vi "pop_dialog.vi"(8 "Property":string[](array[string]), 9 "State In":T2 {"BlockNodeState"."Draw Style" items=["FunctionBlock", "ExpressVI", "Variable", "Elemental I/O", "32x32 Icon", "FunctionBlockCompact"]; "BlockNodeState"."Terminal Data"."Terminal Flags" format="%.0b"}, 10 "FirstTime":bool, 11 "Command Spec":T1) -> (1 "State Out":T2 {"BlockNodeState"."Draw Style" items=["FunctionBlock", "ExpressVI", "Variable", "Elemental I/O", "32x32 Icon", "FunctionBlockCompact"]; "BlockNodeState"."Terminal Data"."Terminal Flags" format="%.0b"}, 2 "NeedUpdate":bool)   [LabVIEW 2018]
uses:
  State.ctl
  <vilib>/BlockNodeSupport/BlockNodeState.ctl
  <vilib>/BlockNodeSupport/TerminalData.ctl
  <vilib>/picture/picture.llb/imagedata.ctl
  command_spec.ctl
  N9010A_SCPI Node.xnode
panel:
  in  "Sort Properties":u16(ring) items=["by Source File Order", "by Property Name", "by SCPI Command"]
  in  "Available Properties Tree":string[](tree)
  in  "Cancel Button":bool
  out "Selected Cmd Pool":string[](array[string])
  out "Available Cmd Pool":string[](array[string])
  in  "Search Within Available Properties":string
  out "Property Help":string
  out "Delete Array":i32[](array[numeric])
  in  "OK Button":bool
  in  "Remove":bool caption="Previous Button"
  in  "Add":bool
  in  "Selected Properties":i32[](listbox)
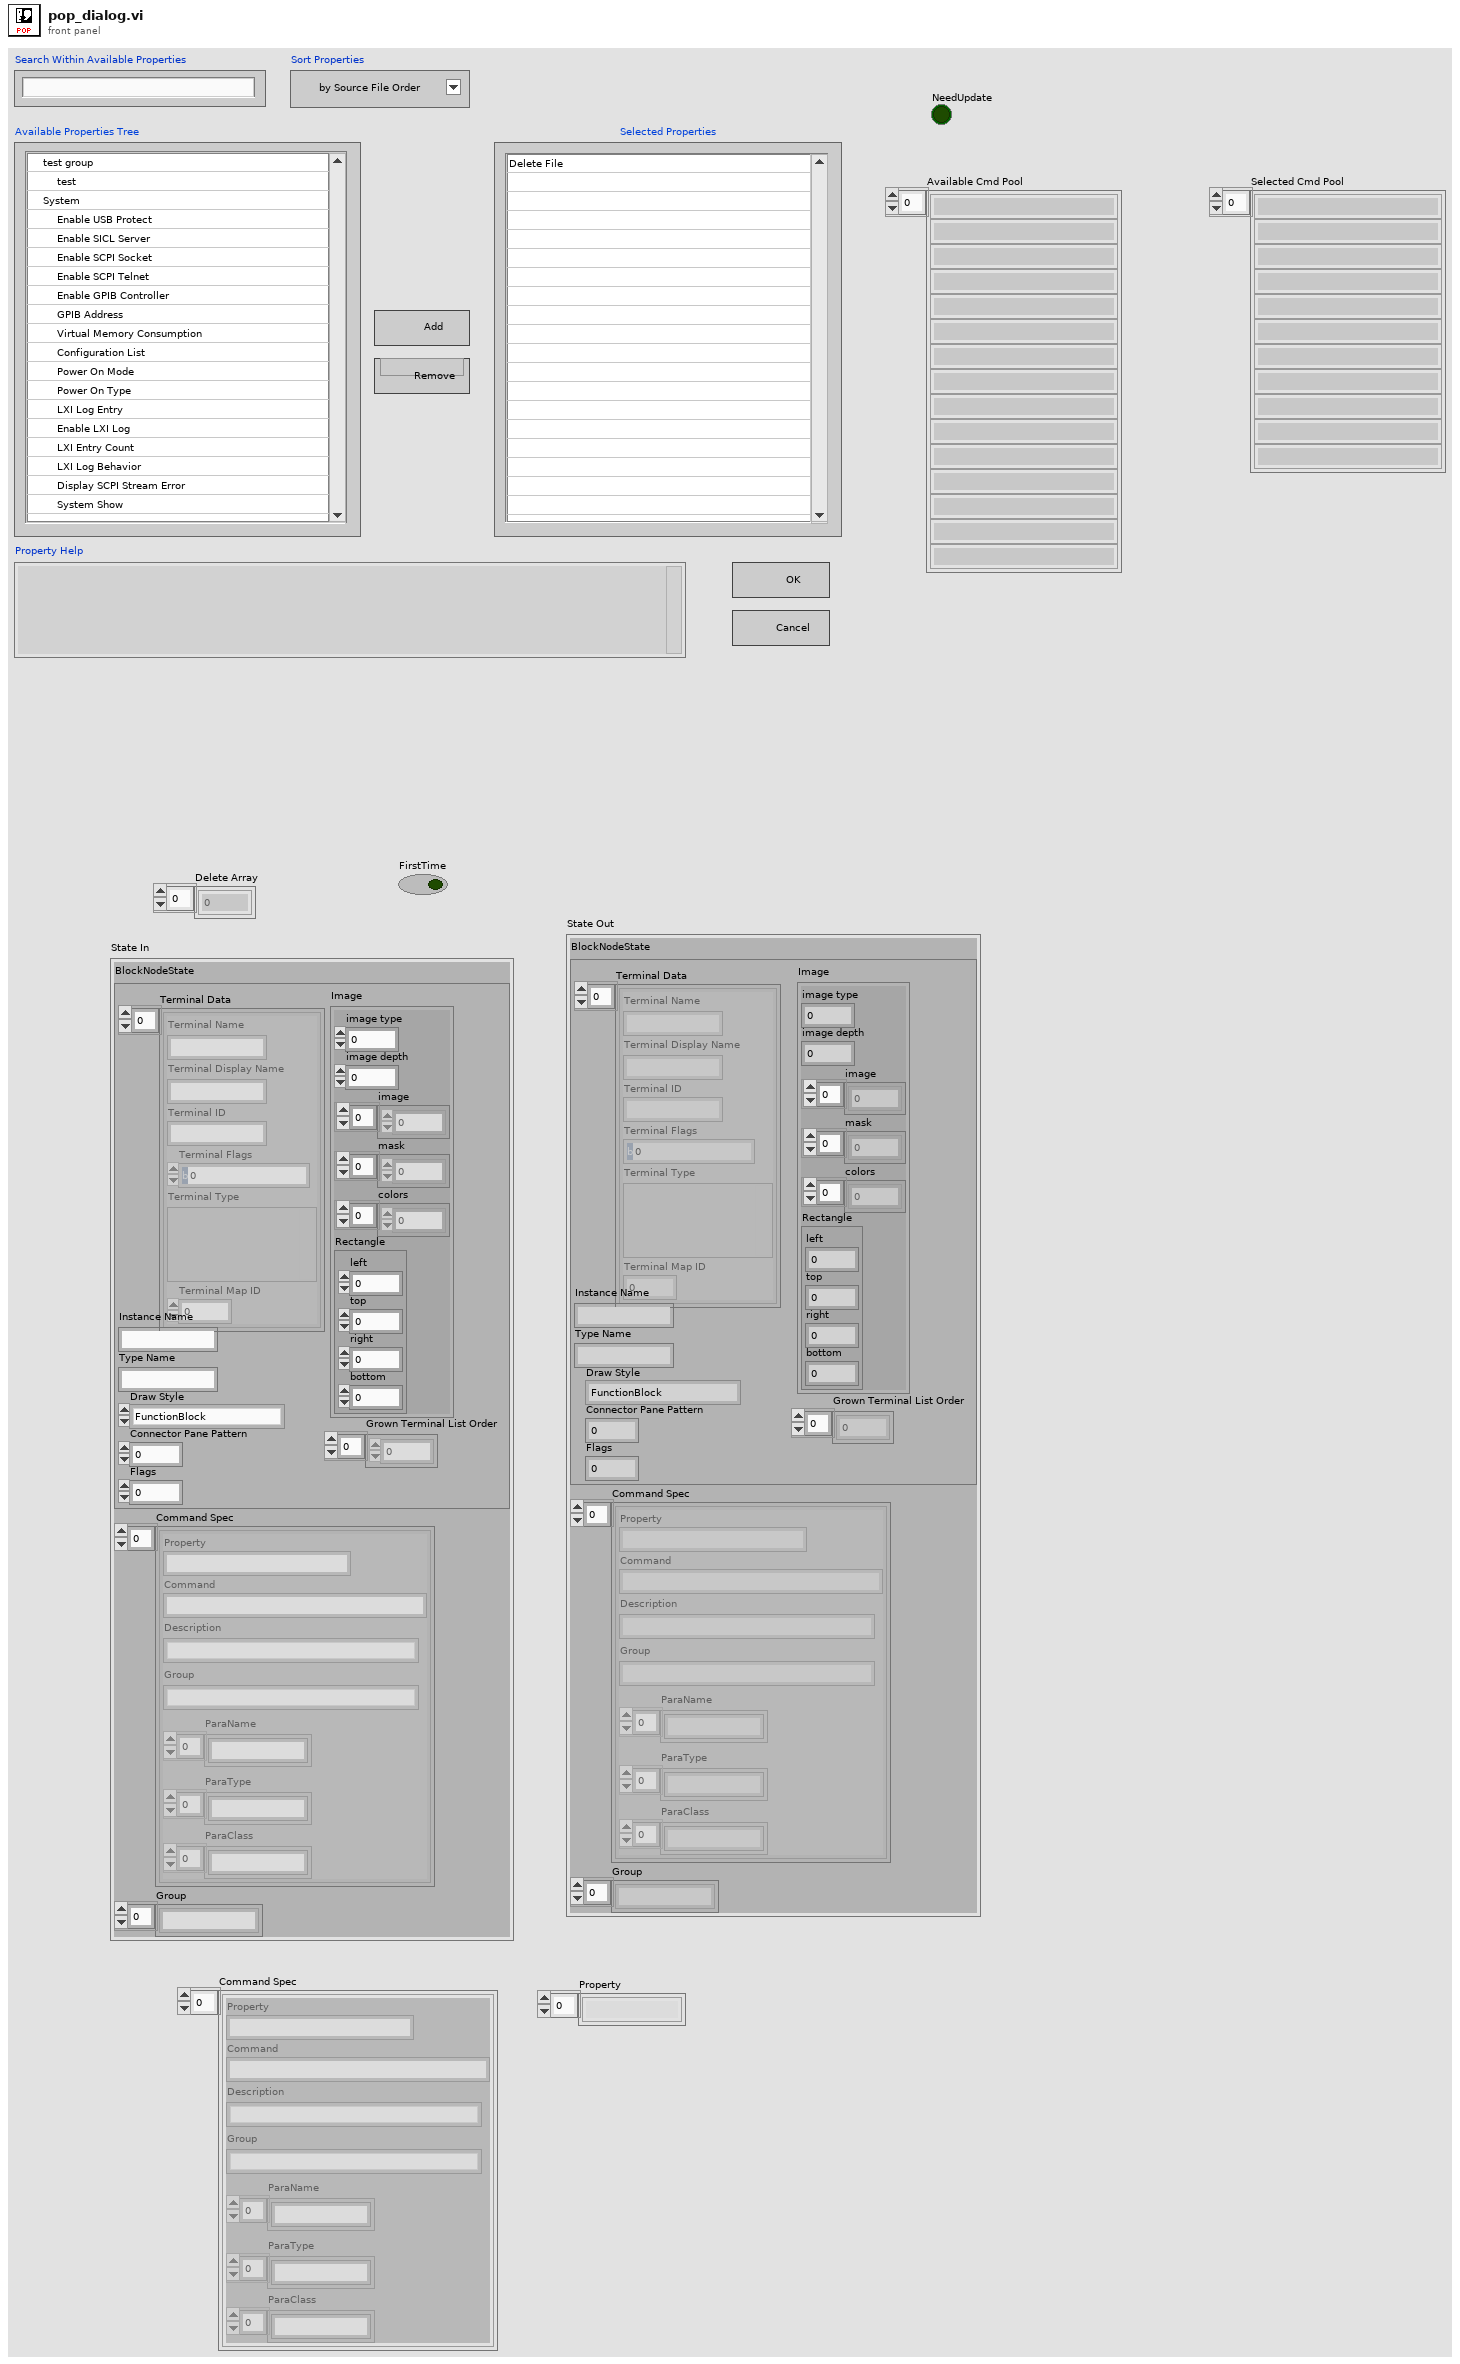
[diagram p1: front panel]
types:
  T1 = typedef "command_spec.ctl" = cluster{"Property":string, "Command":string, "Description":string, "Group":string, "ParaName":string[], "ParaType":string[], "ParaClass":string[]}[]
  T2 = typedef "N9010A_SCPI Node.xnode/State.ctl" = cluster{"BlockNodeState":T3, "Command Spec":T1, "Group":string[]}
  T3 = typedef "BlockNodeState.ctl" = cluster{"Terminal Data":T4[], "Instance Name":string, "Type Name":string, "Draw Style":i32, "Connector Pane Pattern":i32, "Flags":i32, "Grown Terminal List Order":i32[], "Image":T5}
  T4 = typedef "TerminalData.ctl" = cluster{"Terminal Name":string, "Terminal Display Name":string, "Terminal ID":string, "Terminal Flags":i32, "Terminal Type":variant, "Terminal Map ID":i32}
  T5 = typedef "imagedata.ctl" = cluster{"image type":i32, "image depth":i32, "image":u8[], "mask":u8[], "colors":u32[], "Rectangle":cluster{"left":i16, "top":i16, "right":i16, "bottom":i16}}
  T6 = enum8{"Enabled", "Disabled", "Disabled and Grayed Out"}
  T7 = typedef "LVPoint32TypeDef.ctl" = cluster{"Horizontal":i32, "Vertical":i32}
  T8 = cluster{"Property":string, "Command":string, "Description":string, "Group":string, "ParaName":string[], "ParaType":string[], "ParaClass":string[]}
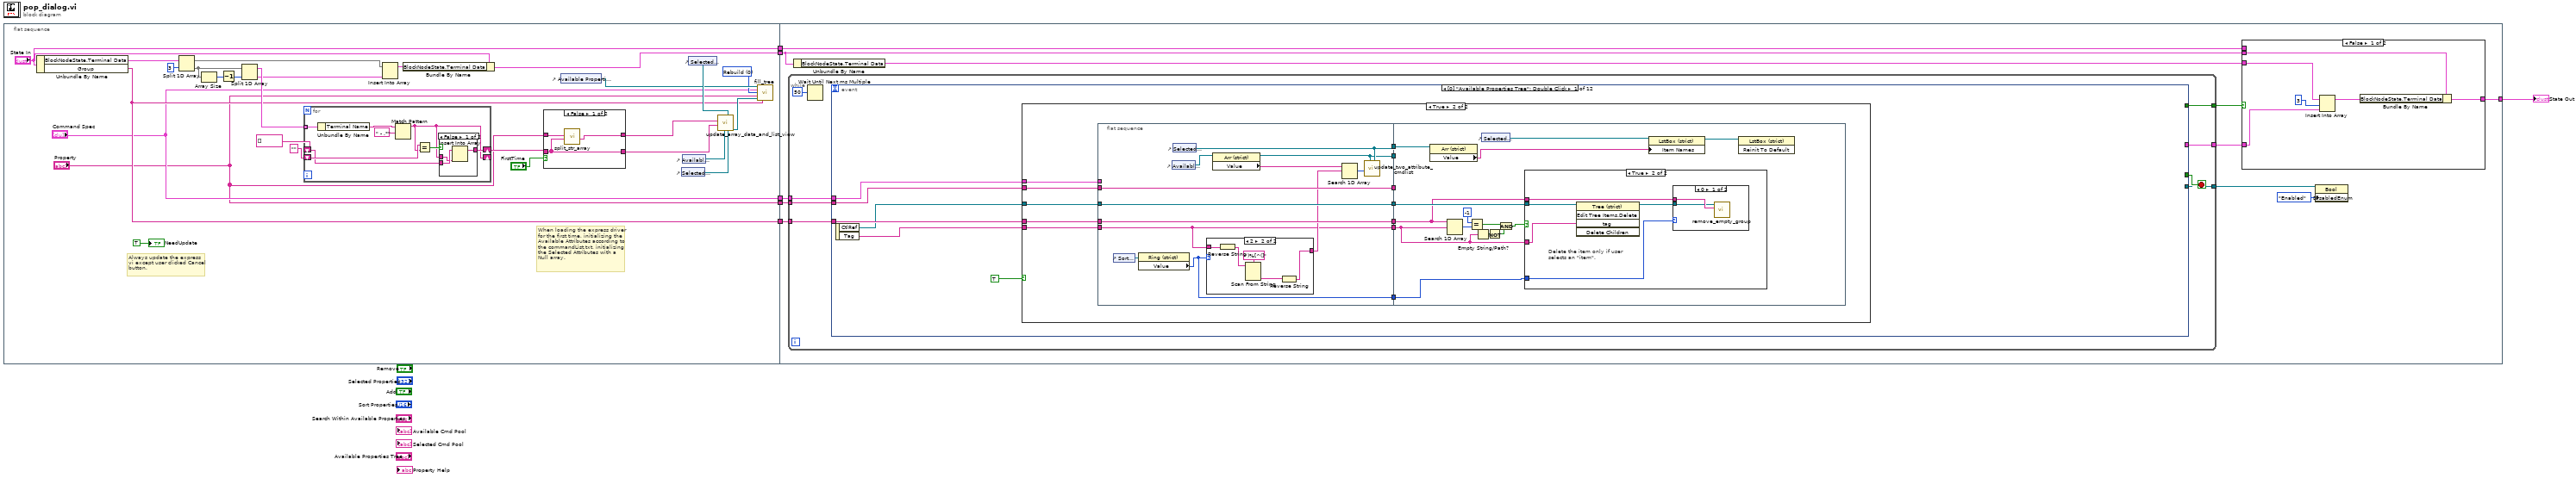
[diagram p0: block diagram]
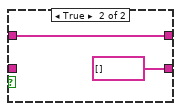
[diagram p2: hidden frame]
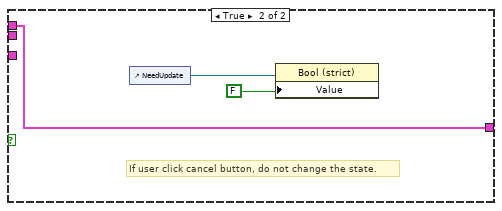
[diagram p4: hidden frame]
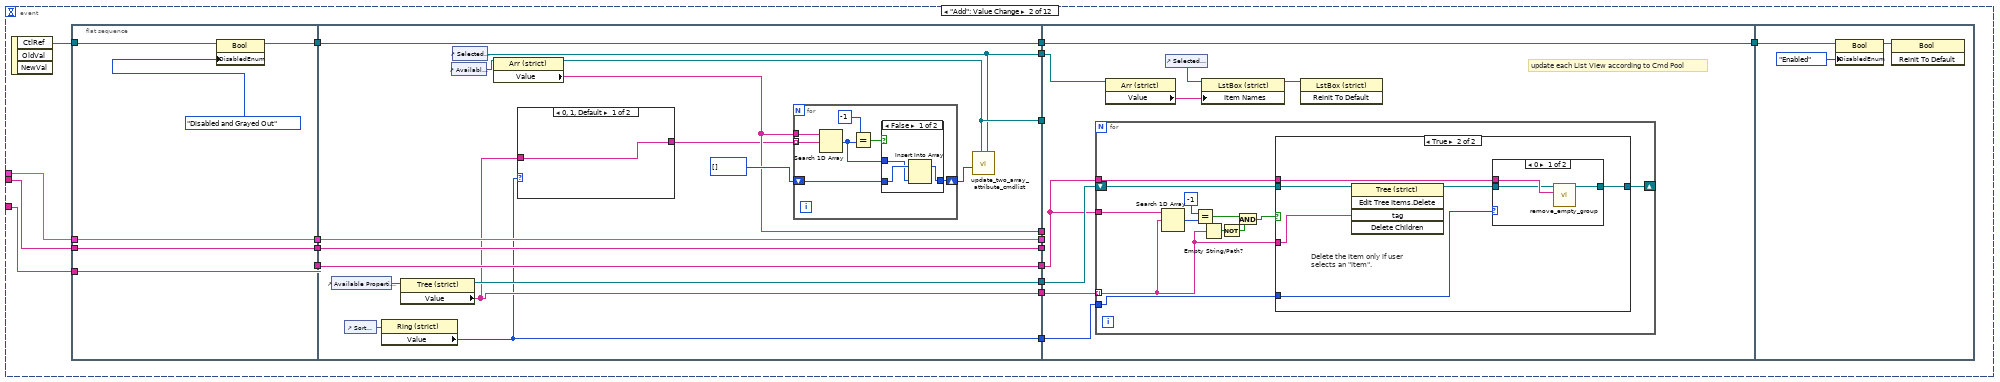
[diagram p9: hidden frame]
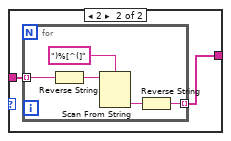
[diagram p10: hidden frame]
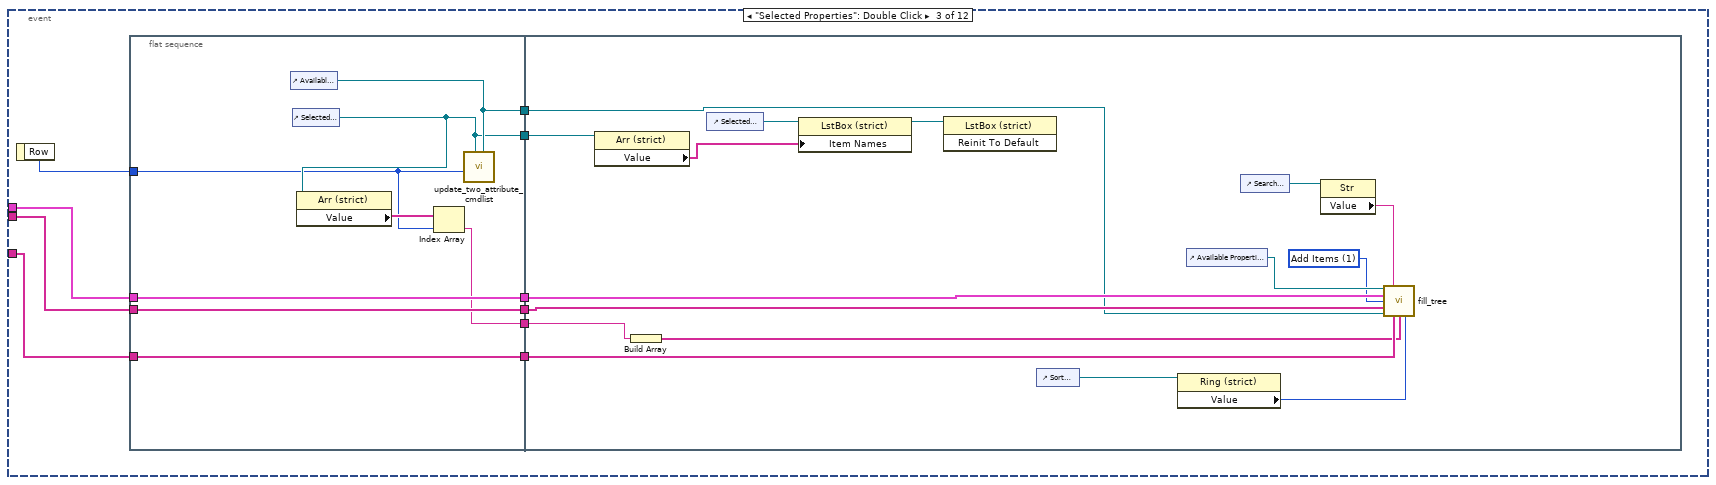
[diagram p14: hidden frame]
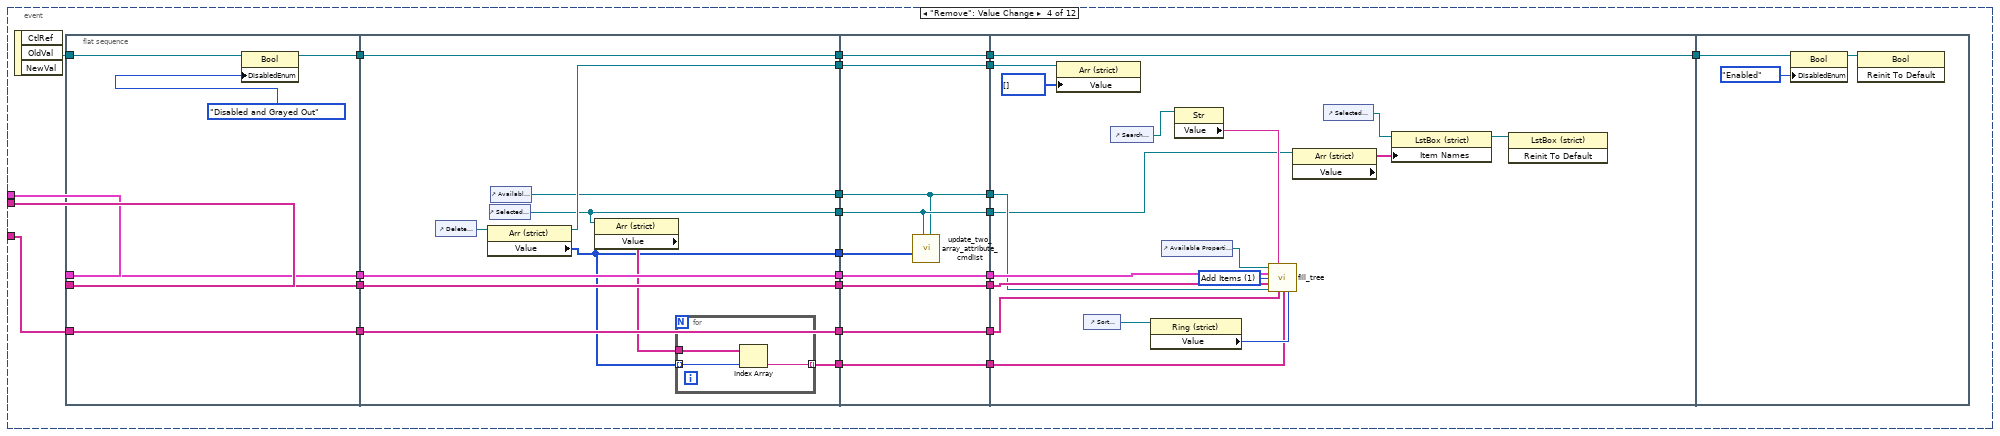
[diagram p15: hidden frame]
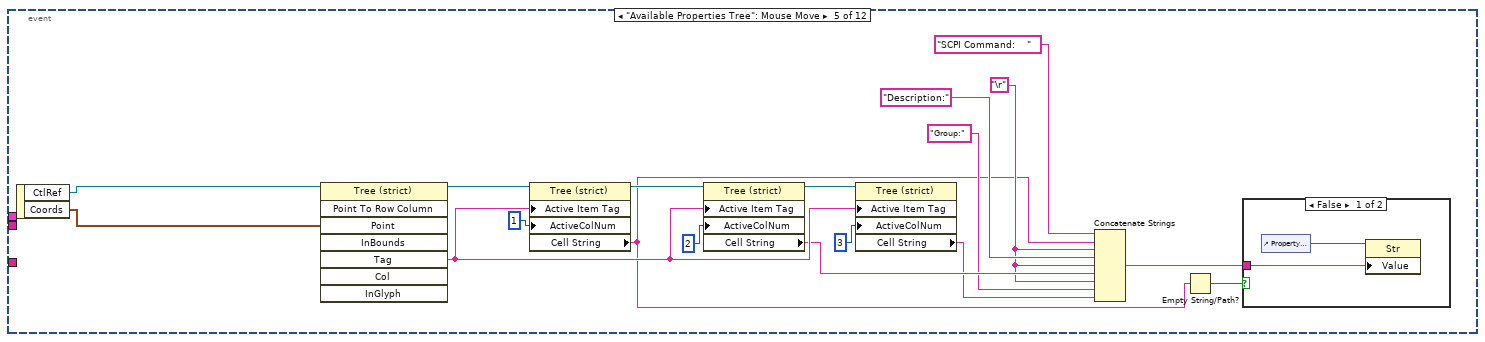
[diagram p16: hidden frame]
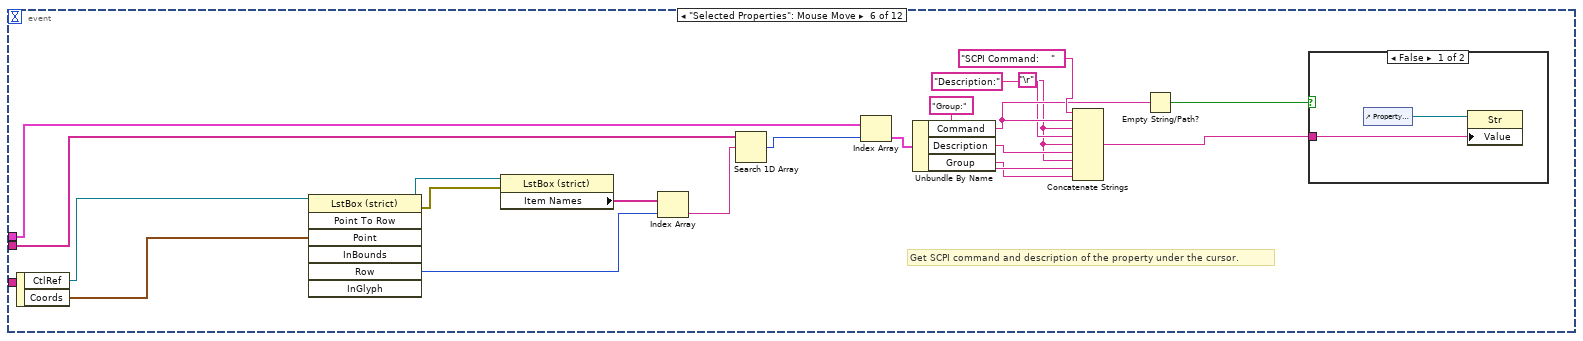
[diagram p18: hidden frame]
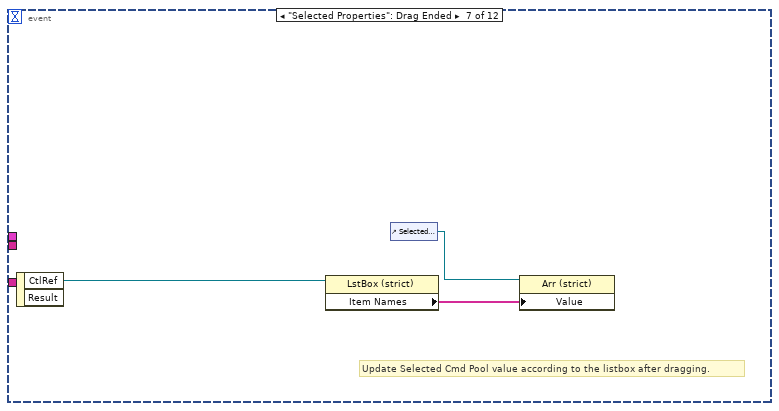
[diagram p20: hidden frame]
diagram:
  n1 = flat-sequence {
    tunnel: ["Command Spec"] -> w6
    tunnel: ["Property"] -> w5
    tunnel: [w32] -> w4
    tunnel: ["State In"] -> w2
    tunnel: [w13] -> w1
    tunnel: w6 -> [w61]
    tunnel: w5 -> [w60]
    tunnel: [w56] -> w3
    tunnel: w4 -> [w57]
    tunnel: w2 -> [w54]
    tunnel: w1 -> [w51]
    frame #0 {
      w9 = u16 0 items=["Rebuild", "Add Single"] ("Operation")
      # "Always update the express\nvi except user clicked Cancel\nbutton."
      # "When loading the express driver\nfor the first time, initializing the\nAvailable Attributes according to\nthe commandList.txt, initializing \nthe Selected Attributes with a\nNull array."
      n2 = Unbundle By Name("State In") -> ("BlockNodeState.Terminal Data"=w31:T4[], "Group"=w13:string[])
      n3 = Split 1D Array(array=w31, index=3) -> (first subarray=w24:T4[], second subarray=w28:T4[])
      n4 = Array Size(array=w28) -> (size(s)=w29:i32)
      n5 = Decrement(x=w29) -> (x-1=w27:i32)
      n6 = Split 1D Array(array=w28, index=w27) -> (first subarray=w26:T4[], second subarray=w25:T4[])
      n7 = for {
        tunnel: w26 -> [w46] mode=indexing
        shift-right: [w40] -> w10
        shift-left: string[] [] ("Array") -> [w41]
        shift-right: [w39] -> _
        shift-left: "" -> [w43]
        n8 = Unbundle By Name(w46) -> ("Terminal Name"=w44:string)
        n9 = Match Pattern(string=w44, regular expression=" - .*") -> (before substring=w39:string)  [unwired: 1 in, 3 out]
        n10 = Equal?(x=w43, y=w39) -> (x = y?=w42:bool)
        n11 = case shown="False" w42 {
          tunnel: w41 -> [w49 w50]
          tunnel: w39 -> [w48 _]
          tunnel: [w47 w50] -> w40
          frame False {
            n12 = Insert Into Array(array=w49, new element=w48) -> (w47:string[])  [unwired: 1 in]
          }
          frame True {
          }
        }
      }
      n13 = Insert Into Array(array=w24, new element=w25) -> (w23:T4[])  [unwired: 1 in]
      n14 = Bundle By Name(cluster="State In", "BlockNodeState.Terminal Data"=w23) -> (w32:T2)
      n15 = case shown="False" "FirstTime" {
        tunnel: "Property" -> [w36 w37]
        tunnel: [w34 string[] [] ("Item Names")] -> w22
        tunnel: [w35 w37] -> w16
        tunnel: w10 -> [w34 _]
        frame False {
          n16 = call "split_str_array.vi"("First  Array"=w34, "Total Array"=w36) -> ("Rest Array"=w35:string[])  [unwired: 9 in]
        }
        frame True {
        }
      }
      n17 = control-ref of="Available Properties Tree"() -> (w15:refnum<vi>)
      n18 = control-ref of="Selected Cmd Pool"() -> (w20:refnum<vi>)
      n19 = control-ref of="Available Cmd Pool"() -> (w21:refnum<vi>)
      n20 = control-ref of="Selected Properties"() -> (w19:refnum<vi>)
      n21 = call "update_array_data_and_list_view.vi"("Cmd Pool 2"=w20, "Cmd Pool 2 List View"=w19, "Cmd Pool 1"=w21, "Cmd Array 2"=w22, "Cmd Array 1"=w16) -> ("Cmd Pool 1 Ref Out"=w14:refnum<vi>)  [unwired: 6 in]
      n22 = call "fill_tree.vi"("Tree Refnum"=w15, "Command Spec"="Command Spec", "Operation"=w9, "Property"="Property", "Available Commands Pool"=w14, "Group"=w13) -> ()  [unwired: 10 in]
      "NeedUpdate" <- TRUE ("NeedUpdate")
    }
    frame #1 {
      n23 = while {
        tunnel: w61 -> [w76]
        tunnel: w60 -> [w77]
        tunnel: [w74] -> w58
        tunnel: [w73] -> w55
        tunnel: [w72] -> w53
        tunnel: w51 -> [w71]
        stop <- w78 stop-if-true
        n24 = Wait Until Next ms Multiple(millisecond multiple=u32 50) -> ()  [unwired: 1 out]
        n25 = event shown="[0] \"Available Properties Tree\": Double Click" {
          selector: _ -> [_ _ _ _ _ _ _ _ _ _ _ _]
          dyn-events: _ -> [_ _ _ _ _ _ _ _ _ _ _ _]
          timeout: _ -> [_ _ _ _ _ _ _ _ _ _ _ _]
          tunnel: [_ _ _ _ _ _ _ _ _ _ w416 "Cancel Button"] -> w78
          tunnel: w77 -> [w82 w147 w234 w287 _ w373 _ _ w391 w406 w414 _]
          tunnel: w76 -> [w83 w148 w236 w286 _ w371 _ _ w392 w407 w415 _]
          tunnel: [_ _ _ _ _ _ _ _ _ _ w412 _] -> w74
          tunnel: [_ _ _ _ _ _ _ _ _ _ _ "Cancel Button"] -> w73
          tunnel: [_ _ _ _ _ _ _ _ _ _ w417 _] -> w72
          tunnel: w71 -> [w84 w140 w233 w283 _ _ _ _ w390 w405 _ _]
          event "Available Properties Tree": Double Click {
            n26 = event-data() -> ("CtlRef"=w80:refnum<vi>, "Tag"=w81:string)  [unwired: 1 in]
            n27 = case shown="True" TRUE {
              tunnel: w84 -> [_ w89]
              tunnel: w83 -> [_ w88]
              tunnel: w82 -> [_ w87]
              tunnel: w81 -> [_ w86]
              tunnel: w80 -> [_ w85]
              frame False {
              }
              frame True {
                n28 = flat-sequence {
                  tunnel: [w106] -> w96
                  tunnel: w86 -> [w98]
                  tunnel: [w98] -> w95
                  tunnel: [w104] -> w94
                  tunnel: w85 -> [w104]
                  tunnel: w89 -> [w103]
                  tunnel: [w103] -> w93
                  tunnel: w88 -> [_]
                  tunnel: [w102] -> w92
                  tunnel: w87 -> [w102]
                  tunnel: [w101] -> w91
                  tunnel: [w97] -> w90
                  tunnel: w96 -> [w124]
                  tunnel: w95 -> [w119]
                  tunnel: w94 -> [w126]
                  tunnel: w93 -> [w121]
                  tunnel: w92 -> [_]
                  tunnel: w91 -> [_]
                  tunnel: w90 -> [w115]
                  frame #0 {
                    n29 = control-ref of="Sort Properties"() -> (w100:refnum<vi>)
                    n30 = property class="Ring (strict)"(reference=w100) -> ("Value"=w97:u16)  [unwired: 1 in, 2 out]
                    n31 = control-ref of="Available Cmd Pool"() -> (w108:refnum<vi>)
                    n32 = control-ref of="Selected Cmd Pool"() -> (w106:refnum<vi>)
                    n33 = case shown="2" w97 {
                      tunnel: w98 -> [w109 w114]
                      tunnel: [w109 w110] -> w99
                      frame 0, 1, Default {
                      }
                      frame 2 {
                        n34 = Reverse String(1:w114) -> (0:w113:string)
                        n35 = Scan From String(format string=")%[^(]", input string=w113) -> (output 1=w111:string)  [unwired: 3 in, 3 out]
                        n36 = Reverse String(1:w111) -> (0:w110:string)
                      }
                    }
                    n37 = property class="Arr (strict)"(reference=w108) -> (reference out=w101:refnum<vi>, "Value"=w105:string[])  [unwired: 1 in, 1 out]
                    n38 = Search 1D Array(1D array=w105, element=w99) -> (index of element=w107:i32)  [unwired: 1 in]
                    n39 = call "update_two_attribute_cmdlist.vi"("Add to Cmd Pool"=w106, "Delete from Cmd Pool"=w101, "Row Index"=w107) -> ()  [unwired: 9 in]
                  }
                  frame #1 {
                    n40 = property class="Arr (strict)"(reference=w124) -> ("Value"=w125:string[])  [unwired: 1 in, 2 out]
                    n41 = Search 1D Array(1D array=w121, element=w119) -> (index of element=w123:i32)  [unwired: 1 in]
                    n42 = Equal?(x=-1, y=w123) -> (x = y?=w118:bool)
                    n43 = Empty String/Path?(string/path=w119) -> (empty?=w117:bool)
                    n44 = control-ref of="Selected Properties"() -> (w128:refnum<vi>)
                    n45 = Not(x=w117) -> (.not. x?=w116:bool)
                    n46 = And(x=w118, y=w116) -> (x .and. y?=w120:bool)
                    n47 = case shown="True" w120 {
                      tunnel: w126 -> [_ w133]
                      tunnel: w119 -> [_ w132]
                      tunnel: w121 -> [_ w131]
                      tunnel: w115 -> [_ w129]
                      frame False {
                      }
                      frame True {
                        # "Delete the item only if user selects an \"item\"."
                        n48 = invoke class="Tree (strict)" method="Edit Tree Items.Delete"(reference=w133, "tag"=w132) -> (reference out=w130:refnum<vi>)  [unwired: 3 in, 4 out]
                        n49 = case shown="0" w129 {
                          tunnel: w131 -> [w135 _]
                          tunnel: w130 -> [w134 _]
                          frame 0 {
                            n50 = call "remove_empty_group.vi"("Group"=w135, "TreeControl In"=w134) -> ()  [unwired: 9 in, 1 out]
                          }
                          frame 1, 2, Default {
                          }
                        }
                      }
                    }
                    n51 = property class="LstBox (strict)"(reference=w128, "Item Names"=w125) -> (reference out=w127:refnum<vi>)  [unwired: 1 in, 1 out]
                    n52 = invoke class="LstBox (strict)" method="Reinit To Default"(reference=w127) -> ()  [unwired: 2 in, 3 out]
                  }
                }
              }
            }
          }
          event "Add": Value Change {
            n53 = event-data() -> ("CtlRef"=w154:refnum<vi>)  [unwired: 1 in, 2 out]
            n54 = flat-sequence {
              tunnel: w154 -> [w160]
              tunnel: [w158] -> w153
              tunnel: w148 -> [w157]
              tunnel: w147 -> [w156]
              tunnel: [w157] -> w145
              tunnel: [w156] -> w143
              tunnel: w140 -> [w155]
              tunnel: [w155] -> w139
              tunnel: w153 -> [w176]
              tunnel: [w176] -> w152
              tunnel: [w172] -> w150
              tunnel: [w171] -> w149
              tunnel: [w170] -> w146
              tunnel: w145 -> [w170]
              tunnel: [w169] -> w144
              tunnel: w143 -> [w169]
              tunnel: [w168] -> w142
              tunnel: [w166] -> w141
              tunnel: w139 -> [w165]
              tunnel: [w165] -> w138
              tunnel: [w162] -> w137
              tunnel: [w161] -> w136
              tunnel: w152 -> [w204]
              tunnel: [w204] -> w151
              tunnel: w150 -> [_]
              tunnel: w149 -> [w201]
              tunnel: w146 -> [_]
              tunnel: w144 -> [_]
              tunnel: w142 -> [_]
              tunnel: w141 -> [w199]
              tunnel: w138 -> [w196]
              tunnel: w137 -> [w198]
              tunnel: w136 -> [w197]
              tunnel: w151 -> [w229]
              frame #0 {
                n55 = property class="Bool"(reference=w160, "DisabledEnum"=T6."Disabled and Grayed Out" ("Disabled")) -> (reference out=w158:refnum<vi>)  [unwired: 1 in, 1 out]
              }
              frame #1 {
                n56 = control-ref of="Available Properties Tree"() -> (w167:refnum<vi>)
                n57 = control-ref of="Sort Properties"() -> (w164:refnum<vi>)
                n58 = property class="Ring (strict)"(reference=w164) -> ("Value"=w161:u16)  [unwired: 1 in, 2 out]
                n59 = property class="Tree (strict)"(reference=w167) -> (reference out=w166:refnum<vi>, "Value"=w162:string[])  [unwired: 1 in, 1 out]
                n60 = control-ref of="Available Cmd Pool"() -> (w175:refnum<vi>)
                n61 = control-ref of="Selected Cmd Pool"() -> (w171:refnum<vi>)
                n62 = property class="Arr (strict)"(reference=w175) -> (reference out=w172:refnum<vi>, "Value"=w168:string[])  [unwired: 1 in, 1 out]
                n63 = case shown="0, 1, Default" w161 {
                  tunnel: w162 -> [w177 w179]
                  tunnel: [w177 w178] -> w163
                  frame 0, 1, Default {
                  }
                  frame 2 {
                    n64 = for {
                      tunnel: w179 -> [w184] mode=indexing
                      tunnel: [w180] -> w178 mode=indexing
                      n65 = Reverse String(1:w184) -> (0:w183:string)
                      n66 = Scan From String(format string=")%[^(]", input string=w183) -> (output 1=w181:string)  [unwired: 3 in, 3 out]
                      n67 = Reverse String(1:w181) -> (0:w180:string)
                    }
                  }
                }
                n68 = for {
                  shift-right: [w186] -> w173
                  shift-left: i32[] [] ("Value") -> [w187]
                  tunnel: w168 -> [w191]
                  tunnel: w163 -> [w190] mode=indexing
                  n69 = Search 1D Array(1D array=w191, element=w190) -> (index of element=w185:i32)  [unwired: 1 in]
                  n70 = Equal?(x=-1, y=w185) -> (x = y?=w188:bool)
                  n71 = case shown="False" w188 {
                    tunnel: w187 -> [w194 w195]
                    tunnel: [w193 w195] -> w186
                    tunnel: w185 -> [w192 _]
                    frame False {
                      n72 = Insert Into Array(array=w194, new element=w192) -> (w193:i32[])  [unwired: 1 in]
                    }
                    frame True {
                    }
                  }
                }
                n73 = call "update_two_array_attribute_cmdlist.vi"("Add to Cmd Pool"=w171, "Delete from Cmd Pool"=w172, "Modified Array"=w173) -> ()  [unwired: 9 in]
              }
              frame #2 {
                # "update each List View according to Cmd Pool"
                n74 = for {
                  tunnel: w196 -> [w210]
                  tunnel: w198 -> [w206] mode=indexing
                  tunnel: w197 -> [w208]
                  shift-right: [w207] -> _
                  shift-left: w199 -> [w209]
                  tunnel: w196 -> [w205]
                  n75 = Search 1D Array(1D array=w205, element=w206) -> (index of element=w216:i32)  [unwired: 1 in]
                  n76 = Equal?(x=-1, y=w216) -> (x = y?=w213:bool)
                  n77 = Empty String/Path?(string/path=w206) -> (empty?=w212:bool)
                  n78 = Not(x=w212) -> (.not. x?=w211:bool)
                  n79 = And(x=w213, y=w211) -> (x .and. y?=w214:bool)
                  n80 = case shown="True" w214 {
                    tunnel: w209 -> [w217 w223]
                    tunnel: w206 -> [_ w222]
                    tunnel: w210 -> [_ w221]
                    tunnel: w208 -> [_ w219]
                    tunnel: [w217 w218] -> w207
                    frame False {
                    }
                    frame True {
                      # "Delete the item only if user selects an \"item\"."
                      n81 = invoke class="Tree (strict)" method="Edit Tree Items.Delete"(reference=w223, "tag"=w222) -> (reference out=w220:refnum<vi>)  [unwired: 3 in, 4 out]
                      n82 = case shown="0" w219 {
                        tunnel: w221 -> [w226 _]
                        tunnel: w220 -> [w225 w227]
                        tunnel: [w224 w227] -> w218
                        frame 0 {
                          n83 = call "remove_empty_group.vi"("Group"=w226, "TreeControl In"=w225) -> ("TreeControl Out"=w224:refnum<vi>)  [unwired: 9 in]
                        }
                        frame 1, 2, Default {
                        }
                      }
                    }
                  }
                }
                n84 = property class="Arr (strict)"(reference=w201) -> ("Value"=w200:string[])  [unwired: 1 in, 2 out]
                n85 = control-ref of="Selected Properties"() -> (w202:refnum<vi>)
                n86 = property class="LstBox (strict)"(reference=w202, "Item Names"=w200) -> (reference out=w203:refnum<vi>)  [unwired: 1 in, 1 out]
                n87 = invoke class="LstBox (strict)" method="Reinit To Default"(reference=w203) -> ()  [unwired: 2 in, 3 out]
              }
              frame #3 {
                n88 = property class="Bool"(reference=w229, "DisabledEnum"=T6."Enabled" ("Disabled")) -> (reference out=w228:refnum<vi>)  [unwired: 1 in, 1 out]
                n89 = invoke class="Bool" method="Reinit To Default"(reference=w228) -> ()  [unwired: 2 in, 3 out]
              }
            }
          }
          event "Selected Properties": Double Click {
            n90 = event-data() -> ("Row"=w240:i32)  [unwired: 1 in]
            n91 = flat-sequence {
              tunnel: w240 -> [w242]
              tunnel: [w248] -> w239
              tunnel: [w244] -> w238
              tunnel: [w247] -> w237
              tunnel: w236 -> [w247]
              tunnel: [w246] -> w235
              tunnel: w234 -> [w246]
              tunnel: w233 -> [w245]
              tunnel: [w245] -> w232
              tunnel: [w241] -> w231
              tunnel: w239 -> [w255]
              tunnel: w238 -> [w253]
              tunnel: w237 -> [w260]
              tunnel: w235 -> [w259]
              tunnel: w232 -> [w258]
              tunnel: w231 -> [w251]
              frame #0 {
                n92 = control-ref of="Available Cmd Pool"() -> (w248:refnum<vi>)
                n93 = control-ref of="Selected Cmd Pool"() -> (w244:refnum<vi>)
                n94 = property class="Arr (strict)"(reference=w244) -> ("Value"=w243:string[])  [unwired: 1 in, 2 out]
                n95 = Index Array(array=w243, index=w242) -> (element=w241:string)
                n96 = call "update_two_attribute_cmdlist.vi"("Add to Cmd Pool"=w248, "Delete from Cmd Pool"=w244, "Row Index"=w242) -> ()  [unwired: 9 in]
              }
              frame #1 {
                w249 = u16 1 items=["Rebuild", "Add Items"] ("Operation")
                n97 = property class="Arr (strict)"(reference=w253) -> ("Value"=w254:string[])  [unwired: 1 in, 2 out]
                n98 = Build Array(w251) -> (w250:string[])
                n99 = control-ref of="Selected Properties"() -> (w262:refnum<vi>)
                n100 = property class="LstBox (strict)"(reference=w262, "Item Names"=w254) -> (reference out=w263:refnum<vi>)  [unwired: 1 in, 1 out]
                n101 = invoke class="LstBox (strict)" method="Reinit To Default"(reference=w263) -> ()  [unwired: 2 in, 3 out]
                n102 = control-ref of="Sort Properties"() -> (w252:refnum<vi>)
                n103 = property class="Ring (strict)"(reference=w252) -> ("Value"=w257:u16)  [unwired: 1 in, 2 out]
                n104 = control-ref of="Available Properties Tree"() -> (w261:refnum<vi>)
                n105 = control-ref of="Search Within Available Properties"() -> (w264:refnum<vi>)
                n106 = property class="Str"(reference=w264) -> ("Value"=w256:string)  [unwired: 1 in, 2 out]
                n107 = call "fill_tree.vi"("Tree Refnum"=w261, "Match String"=w256, "Command Spec"=w260, "Operation"=w249, "Property"=w259, "Available Commands Pool"=w255, "Group"=w258, "Items to Insert"=w250, "Sorting Method"=w257) -> ()  [unwired: 7 in]
              }
            }
          }
          event "Remove": Value Change {
            n108 = event-data() -> ("CtlRef"=w288:refnum<vi>)  [unwired: 1 in, 2 out]
            n109 = flat-sequence {
              tunnel: [w295] -> w290
              tunnel: w288 -> [w294]
              tunnel: w287 -> [w292]
              tunnel: w286 -> [w293]
              tunnel: [w293] -> w285
              tunnel: [w292] -> w284
              tunnel: w283 -> [w291]
              tunnel: [w291] -> w282
              tunnel: w290 -> [w307]
              tunnel: [w307] -> w281
              tunnel: [w306] -> w279
              tunnel: [w304] -> w277
              tunnel: [w300] -> w275
              tunnel: [w303] -> w273
              tunnel: w285 -> [w303]
              tunnel: [w302] -> w271
              tunnel: w284 -> [w302]
              tunnel: [w301] -> w269
              tunnel: w282 -> [w301]
              tunnel: [w298] -> w267
              tunnel: [w297] -> w265
              tunnel: w281 -> [w319]
              tunnel: [w319] -> w280
              tunnel: w279 -> [w318]
              tunnel: [w318] -> w278
              tunnel: w277 -> [w313]
              tunnel: [w313] -> w276
              tunnel: w275 -> [w314]
              tunnel: [w314] -> w274
              tunnel: w273 -> [w317]
              tunnel: [w317] -> w272
              tunnel: w271 -> [w316]
              tunnel: [w316] -> w270
              tunnel: w269 -> [w315]
              tunnel: [w315] -> w268
              tunnel: w267 -> [w312]
              tunnel: [w311] -> w266
              tunnel: w265 -> [w311]
              tunnel: w280 -> [w337]
              tunnel: [w337] -> w289
              tunnel: w278 -> [w336]
              tunnel: w276 -> [w327]
              tunnel: w274 -> [w324]
              tunnel: w272 -> [w329]
              tunnel: w270 -> [w328]
              tunnel: w268 -> [w326]
              tunnel: w266 -> [w321]
              tunnel: w289 -> [w339]
              frame #0 {
                n110 = property class="Bool"(reference=w294, "DisabledEnum"=T6."Disabled and Grayed Out" ("Disabled")) -> (reference out=w295:refnum<vi>)  [unwired: 1 in, 1 out]
              }
              frame #1 {
                n111 = control-ref of="Delete Array"() -> (w305:refnum<vi>)
                n112 = property class="Arr (strict)"(reference=w305) -> (reference out=w306:refnum<vi>, "Value"=w298:i32[])  [unwired: 1 in, 1 out]
                n113 = control-ref of="Selected Cmd Pool"() -> (w300:refnum<vi>)
                n114 = control-ref of="Available Cmd Pool"() -> (w304:refnum<vi>)
                n115 = property class="Arr (strict)"(reference=w300) -> ("Value"=w299:string[])  [unwired: 1 in, 2 out]
                n116 = for {
                  tunnel: w299 -> [w310]
                  tunnel: w298 -> [w309] mode=indexing
                  tunnel: [w308] -> w297 mode=indexing
                  n117 = Index Array(array=w310, index=w309) -> (element=w308:string)
                }
              }
              frame #2 {
                n118 = call "update_two_array_attribute_cmdlist.vi"("Add to Cmd Pool"=w313, "Delete from Cmd Pool"=w314, "Modified Array"=w312) -> ()  [unwired: 9 in]
              }
              frame #3 {
                w320 = u16 1 items=["Rebuild", "Add Items"] ("Operation")
                n119 = property class="Arr (strict)"(reference=w336, "Value"=i32[] []) -> ()  [unwired: 1 in, 2 out]
                n120 = control-ref of="Sort Properties"() -> (w322:refnum<vi>)
                n121 = control-ref of="Search Within Available Properties"() -> (w334:refnum<vi>)
                n122 = property class="Ring (strict)"(reference=w322) -> ("Value"=w325:u16)  [unwired: 1 in, 2 out]
                n123 = control-ref of="Available Properties Tree"() -> (w331:refnum<vi>)
                n124 = property class="Str"(reference=w334) -> ("Value"=w330:string)  [unwired: 1 in, 2 out]
                n125 = call "fill_tree.vi"("Tree Refnum"=w331, "Match String"=w330, "Command Spec"=w329, "Operation"=w320, "Property"=w328, "Available Commands Pool"=w327, "Group"=w326, "Items to Insert"=w321, "Sorting Method"=w325) -> ()  [unwired: 7 in]
                n126 = property class="Arr (strict)"(reference=w324) -> ("Value"=w323:string[])  [unwired: 1 in, 2 out]
                n127 = control-ref of="Selected Properties"() -> (w333:refnum<vi>)
                n128 = property class="LstBox (strict)"(reference=w333, "Item Names"=w323) -> (reference out=w332:refnum<vi>)  [unwired: 1 in, 1 out]
                n129 = invoke class="LstBox (strict)" method="Reinit To Default"(reference=w332) -> ()  [unwired: 2 in, 3 out]
              }
              frame #4 {
                n130 = property class="Bool"(reference=w339, "DisabledEnum"=T6."Enabled" ("Disabled")) -> (reference out=w338:refnum<vi>)  [unwired: 1 in, 1 out]
                n131 = invoke class="Bool" method="Reinit To Default"(reference=w338) -> ()  [unwired: 2 in, 3 out]
              }
            }
          }
          event "Available Properties Tree": Mouse Move {
            w344 = "\r"
            n132 = event-data() -> ("CtlRef"=w357:refnum<vi>, "Coords"=w358:T7)  [unwired: 1 in]
            n133 = invoke class="Tree (strict)" method="Point To Row Column"(reference=w357, "Point"=w358) -> (reference out=w355:refnum<vi>, "Tag"=w350:string)  [unwired: 6 in, 6 out]
            n134 = property class="Tree (strict)"(reference=w355, "Active Item Tag"=w350, "ActiveColNum"=1 ("Active Cell:Active Column Number")) -> (reference out=w352:refnum<vi>, "Cell String"=w343:string)  [unwired: 1 in, 1 out]
            n135 = property class="Tree (strict)"(reference=w352, "Active Item Tag"=w350, "ActiveColNum"=2 ("Active Cell:Active Column Number")) -> (reference out=w351:refnum<vi>, "Cell String"=w347:string)  [unwired: 1 in, 1 out]
            n136 = property class="Tree (strict)"(reference=w351, "Active Item Tag"=w350, "ActiveColNum"=3 ("Active Cell:Active Column Number")) -> ("Cell String"=w346:string)  [unwired: 1 in, 2 out]
            n137 = Concatenate Strings("SCPI Command:    " ("string"), w343, w344, "Description:" ("string"), w344, w347, w344, "Group:" ("string"), w346) -> (w342:string)
            n138 = Empty String/Path?(string/path=w343) -> (empty?=w341:bool)
            n139 = case shown="False" w341 {
              tunnel: w342 -> [w359 _]
              frame False {
                n140 = control-ref of="Property Help"() -> (w360:refnum<vi>)
                n141 = property class="Str"(reference=w360, "Value"=w359) -> ()  [unwired: 1 in, 2 out]
              }
              frame True {
              }
            }
          }
          event "Selected Properties": Mouse Move {
            w362 = "\r"
            # "Get SCPI command and description of the property under the cursor."
            n142 = event-data() -> ("CtlRef"=w379:refnum<vi>, "Coords"=w380:T7)  [unwired: 1 in]
            n143 = invoke class="LstBox (strict)" method="Point To Row"(reference=w379, "Point"=w380) -> (reference out=w378:refnum<vi>, error out=w377:errorcluster, "Row"=w375:i32)  [unwired: 5 in, 4 out]
            n144 = property class="LstBox (strict)"(reference=w378, error in=w377) -> ("Item Names"=w376:string[])  [unwired: 2 out]
            n145 = Index Array(array=w376, index=w375) -> (element=w374:string)
            n146 = Search 1D Array(1D array=w373, element=w374) -> (index of element=w372:i32)  [unwired: 1 in]
            n147 = Index Array(array=w371, index=w372) -> (element=w370:T8)
            n148 = Unbundle By Name(w370) -> ("Command"=w368:string, "Description"=w364:string, "Group"=w361:string)
            n149 = Concatenate Strings("SCPI Command:    " ("string"), w368, w362, "Description:" ("string"), w362, w364, w362, "Group:" ("string"), w361) -> (w366:string)
            n150 = Empty String/Path?(string/path=w368) -> (empty?=w367:bool)
            n151 = case shown="False" w367 {
              tunnel: w366 -> [w381 _]
              frame False {
                n152 = control-ref of="Property Help"() -> (w382:refnum<vi>)
                n153 = property class="Str"(reference=w382, "Value"=w381) -> ()  [unwired: 1 in, 2 out]
              }
              frame True {
              }
            }
          }
          event "Selected Properties": Drag Ended {
            # "Update Selected Cmd Pool value according to the listbox after dragging."
            n154 = event-data() -> ("CtlRef"=w385:refnum<vi>)  [unwired: 1 in, 1 out]
            n155 = property class="LstBox (strict)"(reference=w385) -> ("Item Names"=w383:string[])  [unwired: 1 in, 2 out]
            n156 = control-ref of="Selected Cmd Pool"() -> (w384:refnum<vi>)
            n157 = property class="Arr (strict)"(reference=w384, "Value"=w383) -> ()  [unwired: 1 in, 2 out]
          }
          event "Selected Properties": Value Change {
            n158 = event-data() -> ("NewVal"=→"Delete Array":i32[])  [unwired: 1 in, 2 out]
          }
          event "Search Within Available Properties": Value Change {
            n159 = event-data() -> ("OldVal"=w389:string, "NewVal"=w388:string)  [unwired: 1 in, 1 out]
            n160 = Not Equal?(x=w389, y=w388) -> (x != y?=w387:bool)
            n161 = case shown="True" w387 {
              tunnel: w392 -> [_ w399]
              tunnel: w391 -> [_ w398]
              tunnel: w390 -> [_ w397]
              tunnel: w388 -> [_ w395]
              frame False {
              }
              frame True {
                n162 = control-ref of="Sort Properties"() -> (w393:refnum<vi>)
                n163 = control-ref of="Available Cmd Pool"() -> (w396:refnum<vi>)
                n164 = property class="Ring (strict)"(reference=w393) -> ("Value"=w394:u16)  [unwired: 1 in, 2 out]
                n165 = control-ref of="Available Properties Tree"() -> (w400:refnum<vi>)
                n166 = call "fill_tree.vi"("Tree Refnum"=w400, "Match String"=w395, "Command Spec"=w399, "Property"=w398, "Available Commands Pool"=w396, "Group"=w397, "Sorting Method"=w394) -> ()  [unwired: 9 in]
              }
            }
          }
          event "Sort Properties": Value Change {
            n167 = event-data() -> ("NewVal"=w408:u16)  [unwired: 1 in, 2 out]
            n168 = control-ref of="Available Cmd Pool"() -> (w402:refnum<vi>)
            n169 = control-ref of="Available Properties Tree"() -> (w403:refnum<vi>)
            n170 = control-ref of="Search Within Available Properties"() -> (w404:refnum<vi>)
            n171 = property class="Str"(reference=w404) -> ("Value"=w401:string)  [unwired: 1 in, 2 out]
            n172 = call "fill_tree.vi"("Tree Refnum"=w403, "Match String"=w401, "Command Spec"=w407, "Property"=w406, "Available Commands Pool"=w402, "Group"=w405, "Sorting Method"=w408) -> ()  [unwired: 9 in]
          }
          event "OK Button": Value Change {
            n173 = event-data() -> ("CtlRef"=w418:refnum<vi>)  [unwired: 1 in]
            n174 = control-ref of="Selected Cmd Pool"() -> (w419:refnum<vi>)
            n175 = property class="Arr (strict)"(reference=w419) -> ("Value"=w413:string[])  [unwired: 1 in, 2 out]
            n176 = for {
              tunnel: [w445] -> w411 mode=indexing
              tunnel: w415 -> [w444]
              tunnel: w414 -> [w443]
              tunnel: w413 -> [w442] mode=indexing
              n177 = Search 1D Array(1D array=w443, element=w442) -> (index of element=w446:i32)  [unwired: 1 in]
              n178 = Index Array(array=w444, index=w446) -> (element=w445:T8)
            }
            n179 = for {
              tunnel: w411 -> [w424] mode=indexing
              shift-right: [w420] -> w409
              shift-left: 0 -> [w421]
              n180 = Unbundle By Name(w424) -> ("ParaName"=w423:string[])
              n181 = Array Size(array=w423) -> (size(s)=w422:i32)
              n182 = Add(x=w422, y=w421) -> (x+y=w420:i32)
            }
            n183 = case shown="9.., Default" w409 {
              tunnel: w418 -> [w427 w441]
              tunnel: [w426 w440] -> w417
              tunnel: [FALSE ("OK Button") "OK Button"] -> w416
              tunnel: [T4[] [] ("Block Data Array") w438] -> w412
              tunnel: w411 -> [_ w433]
              frame 9.., Default {
                n184 = invoke class="Bool" method="Reinit To Default"(reference=w427) -> (reference out=w426:refnum<vi>)  [unwired: 2 in, 2 out]
                n185 = One Button Dialog(message="You cannot select properties which contain more than 8 parameters in total.\nPlease remove some properties from \"Selected Properties\".") -> ()  [unwired: 1 in, 1 out]
              }
              frame 0..8 {
                # "Reinit the search control and sort control."
                n186 = Current VI's Path() -> (path=w430:path)
                n187 = Build Path(base path=w430, name or relative path="..\\auto_gen_logic.vi") -> (appended path=w432:path)
                n188 = call "gen_logic_vi_with_cmd_array.vi"("CmdInfo"=w433, "VI Paths"=w432) -> ("VI Paths Out"=w434:path)  [unwired: 9 in]
                n189 = control-ref of="Sort Properties"() -> (w437:refnum<vi>)
                n190 = control-ref of="Search Within Available Properties"() -> (w436:refnum<vi>)
                n191 = call "generate_block_data_array.vi"("VI Paths"=w434) -> ("Block Data Array"=w438:T4[])  [unwired: 10 in]
                n192 = invoke class="Ring (strict)" method="Reinit To Default"(reference=w437) -> ()  [unwired: 2 in, 3 out]
                n193 = invoke class="Str" method="Reinit To Default"(reference=w436) -> ()  [unwired: 2 in, 3 out]
                n194 = property class="Bool"(reference=w441, "DisabledEnum"=T6."Disabled and Grayed Out" ("Disabled")) -> (reference out=w440:refnum<vi>)  [unwired: 1 in, 1 out]
              }
            }
          }
          event "Cancel Button": Value Change {
            # "Reinit the search control and sort control."
            n195 = event-data() -> ()  [unwired: 1 in, 3 out]
            n196 = control-ref of="Sort Properties"() -> (w447:refnum<vi>)
            n197 = control-ref of="Search Within Available Properties"() -> (w448:refnum<vi>)
            n198 = invoke class="Ring (strict)" method="Reinit To Default"(reference=w447) -> ()  [unwired: 2 in, 3 out]
            n199 = invoke class="Str" method="Reinit To Default"(reference=w448) -> ()  [unwired: 2 in, 3 out]
          }
        }
      }
      n200 = Unbundle By Name(w57) -> ("BlockNodeState.Terminal Data"=w59:T4[])
      n201 = case shown="False" w55 {
        tunnel: w59 -> [w66 _]
        tunnel: w58 -> [w65 _]
        tunnel: w57 -> [w64 _]
        tunnel: [w63 w70] -> w56
        tunnel: w54 -> [_ w70]
        frame False {
          n202 = Insert Into Array(array=w66, index=3, new element=w65) -> (w62:T4[])
          n203 = Bundle By Name(cluster=w64, "BlockNodeState.Terminal Data"=w62) -> (w63:T2)
        }
        frame True {
          # "If user click cancel button, do not change the state."
          n204 = control-ref of="NeedUpdate"() -> (w68:refnum<vi>)
          n205 = property class="Bool (strict)"(reference=w68, "Value"=FALSE) -> ()  [unwired: 1 in, 2 out]
        }
      }
      n206 = property class="Bool"(reference=w53, "DisabledEnum"=T6."Enabled" ("Disabled")) -> ()  [unwired: 1 in, 2 out]
    }
  }
  "State Out" <- w3
